vi "Auto-Write to Folder and file for Stuckbead Scan_YCC.vi"(5 "Axis (Enum)":enum16{"x", "y", "z"}(ring), 6 "data to be saved":dbl[][](array[numeric]) format="%0.2f", 7 "Who's Data":T1(ring), 8 "File name add to the end":string="h300", 9 "Save?":bool) -> (2 "Save to File Name":string, 3 "Save to Path":path)   [LabVIEW 2014]
uses:
  Main-Stage-Based/(Global) Current handle and LaserPower_YCC.vi
  <vilib>/Utility/file.llb/Write To Spreadsheet File (DBL).vi
panel:
  out "Folder name":string
  out "folder exists?":bool
  out "date/time string":string
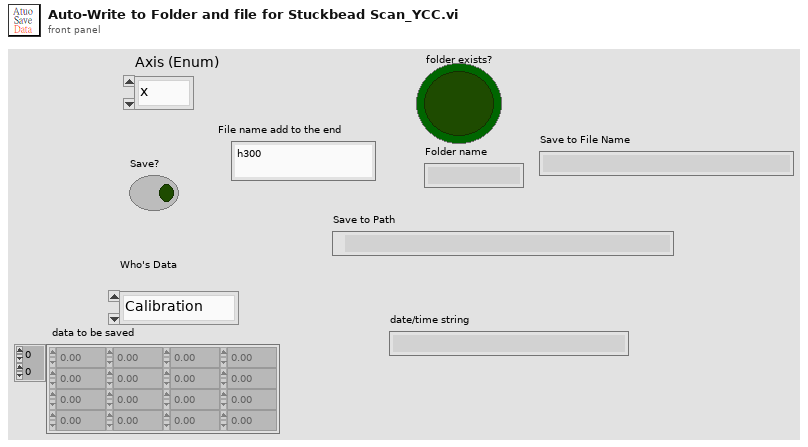
[diagram p1: front panel]
types:
  T1 = enum16{"Calibration", "YCC", "PYW", "LCH", "YYH"}
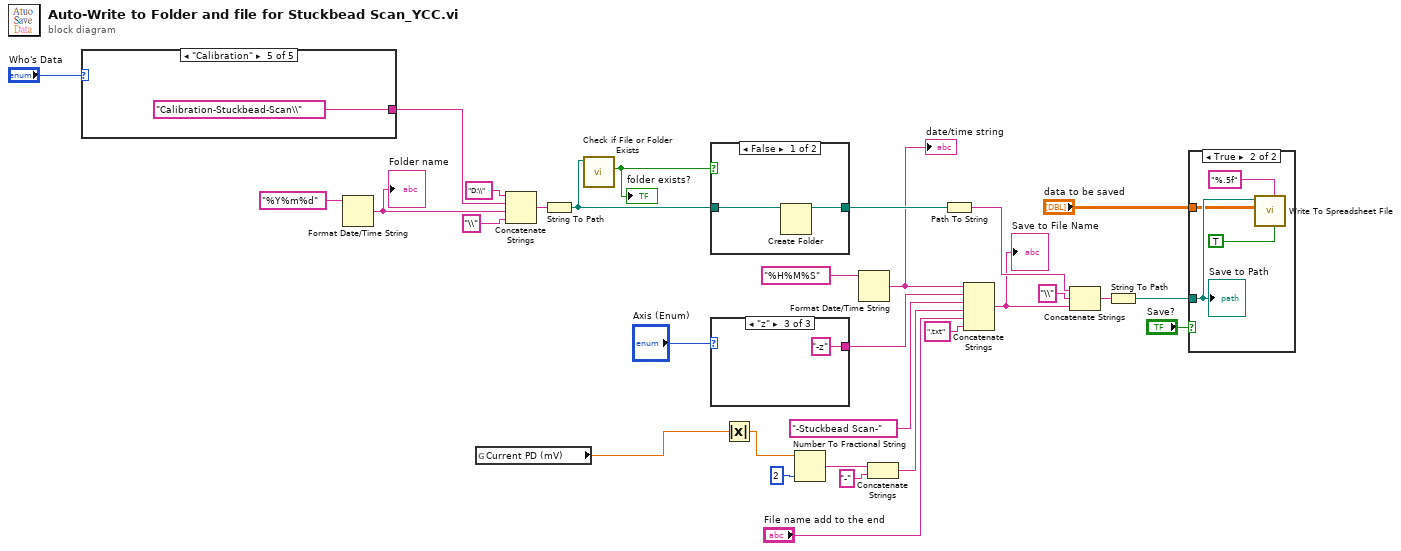
[diagram p0: block diagram]
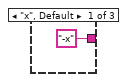
[diagram p2: hidden frame]
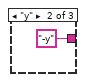
[diagram p3: hidden frame]
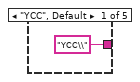
[diagram p6: hidden frame]
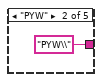
[diagram p7: hidden frame]
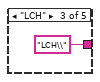
[diagram p8: hidden frame]
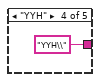
[diagram p9: hidden frame]
diagram:
  n1 = case shown="\"Calibration\"" "Who's Data" {
    tunnel: ["YCC\\" ("string") "PYW\\" ("string") "LCH\\" ("string") "YYH\\" ("string") "Calibration-Stuckbead-Scan\\" ("string")] -> w28
    frame "YCC", Default {
    }
    frame "PYW" {
    }
    frame "LCH" {
    }
    frame "YYH" {
    }
    frame "Calibration" {
    }
  }
  n2 = Format Date/Time String(time format string (%c)="%Y%m%d") -> (date/time string=w15:string)  [unwired: 2 in]
  "Folder name" <- w15
  n3 = global read "(Global) Current handle and LaserPower_YCC.vi" "Current PD (mV)"() -> (w2:dbl)
  n4 = Concatenate Strings("D:\\" ("string"), w28, w15, "\\" ("string")) -> (w27:string)
  n5 = String To Path(string=w27) -> (path=w18:path)
  n6 = call <vilib>:"Check if File or Folder Exists.vi"("path"=w18) -> ("file or folder exists?"=w17:bool)  [unwired: 8 in, 2 out]
  "folder exists?" <- w17
  n7 = case shown="False" w17 {
    tunnel: w18 -> [w37 w38]
    tunnel: [w36 w38] -> w23
    frame False {
      n8 = Create Folder(path (use dialog)=w37) -> (created path=w36:path)  [unwired: 2 in, 2 out]
    }
    frame True {
    }
  }
  n9 = case shown="\"z\"" "Axis (Enum)" {
    tunnel: ["-x" ("string") "-y" ("string") "-z" ("string")] -> w3
    frame "x", Default {
    }
    frame "y" {
    }
    frame "z" {
    }
  }
  n10 = Absolute Value(x=w2) -> (abs(x)=w1:dbl)
  n11 = Number To Fractional String(number=w1, precision (6)=i16 2) -> (F-format string=w9:string)  [unwired: 2 in]
  n12 = Format Date/Time String(time format string (%c)="%H%M%S") -> (date/time string=w5:string)  [unwired: 2 in]
  "date/time string" <- w5
  n13 = Concatenate Strings(w9, "-" ("string")) -> (w7:string)
  n14 = Path To String(path=w23) -> (string=w20:string)
  n15 = Concatenate Strings(w5, w3, "-Stuckbead Scan-" ("string"), w7, "File name add to the end", ".txt" ("string")) -> (w14:string)
  "Save to File Name" <- w14
  n16 = Concatenate Strings(w20, "\\" ("string"), w14) -> (w22:string)
  n17 = String To Path(string=w22) -> (path=w21:path)
  n18 = case shown="True" "Save?" {
    tunnel: w21 -> [_ w44]
    tunnel: "data to be saved" -> [_ w43]
    frame False {
    }
    frame True {
      n19 = call-poly <vilib>:"Write To Spreadsheet File.vi"("transpose? (no:F)"=TRUE, "format (%.3f)"="%.5f", "2D data"=w43, "file path (dialog if empty)"=w44) -> ()  [unwired: 4 in, 1 out]
      "Save to Path" <- w44
    }
  }
